vi "Init.vi"(8 "error in (no error)":errorcluster, 11 "NEO480HTA Base CFG in":refnum<class "Read All CFG.lvclass">) -> (0 "error out":errorcluster, 3 "NEO480HTA Base CFG out":refnum<class "Read All CFG.lvclass">)   [LabVIEW 2023, in "NEO480HTA.lvlib" / "Read All CFG.lvclass"]
uses:
  Read All CFG.lvclass
  <vilib>/Utility/error.llb/Error Cluster From Error Code.vi
  <vilib>/ErrorRing/Error Ring.xnode
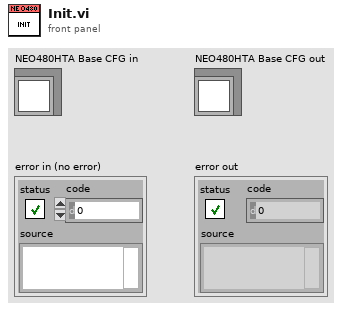
[diagram p1: front panel]
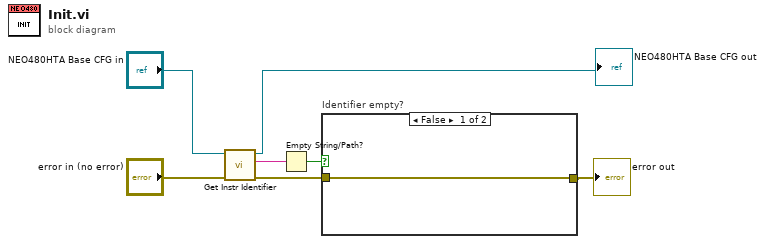
[diagram p0: block diagram]
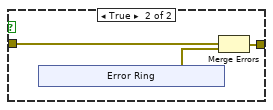
[diagram p2: hidden frame]
diagram:
  n1 = call-dynamic "Get Instr Identifier.vi"("error in (no error)"="error in (no error)", "Configuration Base in"="NEO480HTA Base CFG in") -> ("error out"=w4:errorcluster, "Instr Identifier"=w1:string, "Configuration Base out"=→"NEO480HTA Base CFG out":refnum<class "Read All CFG.lvclass">)  [unwired: 7 in]
  n2 = Empty String/Path?(string/path=w1) -> (empty?=w2:bool)
  n3 = case "Identifier empty?" shown="False" w2 {
    tunnel: w4 -> [w8 w11]
    tunnel: [w8 w10] -> w3
    frame False {
    }
    frame True {
      n4 = xnode "Error Ring"() -> ("error out"=w9:errorcluster)
      n5 = Merge Errors(w11, w9) -> (w10:errorcluster)
    }
  }
  "error out" <- w3
